vi "LVClass_WavefrontCorrectorSet Get Files Destination.vi"(0 "WavefrontCorrectorSet in":refnum<class "WavefrontCorrectorSet.lvclass">, 5 "Folder":path, 11 "error in (no error)":errorcluster) -> (4 "WavefrontCorrectorSet out":refnum<class "WavefrontCorrectorSet.lvclass">, 15 "error out":errorcluster)   [LabVIEW 2020, in "WavefrontCorrectorSet.lvclass"]
uses:
  WavefrontCorrectorSet.lvclass
  WavefrontCorrectorSet.lvclass/WavefrontCorrectorSet.ctl
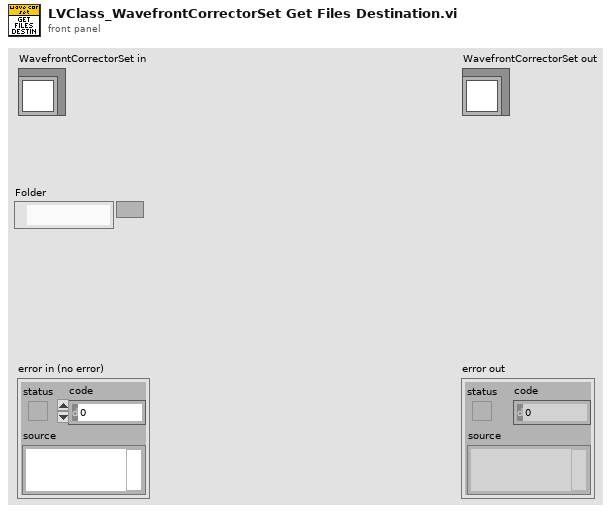
[diagram p1: front panel]
types:
  T1 = typedef "WavefrontCorrectorSpecifications.ctl" = cluster{"Mirror name":string, "Plugin name":string, "Serial number":string, "Revision":string, "Number of commands":i32, "Sleep after command apply (ms)":i32, "Has internal memory ?":bool}
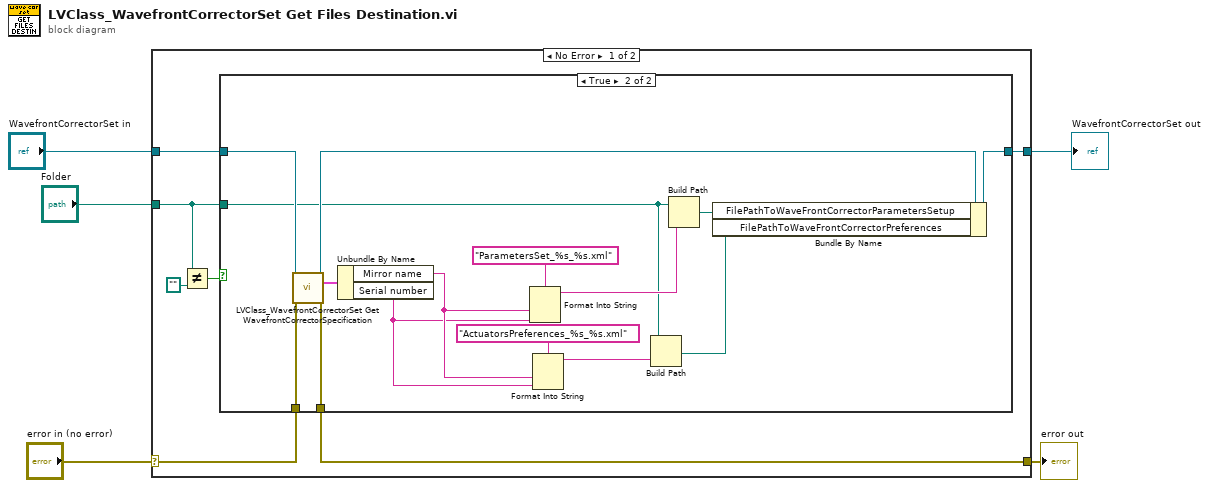
[diagram p0: block diagram]
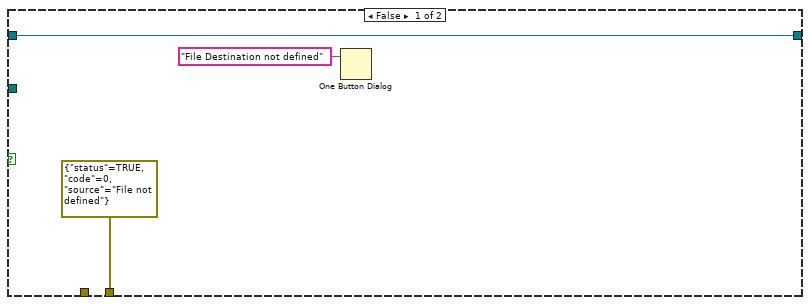
[diagram p2: hidden frame]
diagram:
  n1 = case shown="No Error" "error in (no error)" {
    selector: "error in (no error)" -> [w12 w32]
    tunnel: [w11 w32] -> w4
    tunnel: [w9 w31] -> w2
    tunnel: "WavefrontCorrectorSet in" -> [w10 w31]
    tunnel: "Folder" -> [w6 _]
    frame No Error {
      n2 = Not Equal?(x=w6, y=path "") -> (x != y?=w7:bool)
      n3 = case shown="True" w7 {
        tunnel: w12 -> [_ w26]
        tunnel: [errorcluster {"status"=TRUE, "code"=0, "source"="File not defined"} ("error out") w25] -> w11
        tunnel: w10 -> [w13 w27]
        tunnel: w6 -> [_ w19]
        tunnel: [w13 w30] -> w9
        frame False {
          n4 = One Button Dialog(message="File Destination not defined") -> ()  [unwired: 1 in, 1 out]
        }
        frame True {
          n5 = call "LVClass_WavefrontCorrectorSet Get WavefrontCorrectorSpecification.vi"("WavefrontCorrectorSet in"=w27, "error in (no error)"=w26) -> ("WavefrontCorrectorSet out"=w24:refnum<class "WavefrontCorrectorSet.lvclass">, "ConfigMiroir"=w23:T1, "error out"=w25:errorcluster)  [unwired: 11 in]
          n6 = Unbundle By Name(w23) -> ("Mirror name"=w22:string, "Serial number"=w21:string)
          n7 = Format Into String(format string="ParametersSet_%s_%s.xml", w22, w21) -> (resulting string=w28:string)  [unwired: 2 in, 1 out]
          n8 = Format Into String(format string="ActuatorsPreferences_%s_%s.xml", w22, w21) -> (resulting string=w20:string)  [unwired: 2 in, 1 out]
          n9 = Build Path(base path=w19, name or relative path=w20) -> (appended path=w18:path)
          n10 = Build Path(base path=w19, name or relative path=w28) -> (appended path=w17:path)
          n11 = Bundle By Name(cluster=w24, "FilePathToWaveFrontCorrectorParametersSetup"=w17, "FilePathToWaveFrontCorrectorPreferences"=w18) -> (w30:refnum<class "WavefrontCorrectorSet.lvclass">)
        }
      }
    }
    frame Error {
    }
  }
  "error out" <- w4
  "WavefrontCorrectorSet out" <- w2
